vi "BodeMagnitudePlot.vi"() -> ()   [LabVIEW 2014]
uses:
  <vilib>/Analysis/NI_AALPro.lvlib
panel:
  out "XY Graph":cluster{i32, "AC estimate (Vrms)":dbl}[](graph)=[{10, "AC estimate (Vrms)"=-0.004675753198457834}, {35, "AC estimate (Vrms)"=-0.0035149121931835688}, {60, "AC estimate (Vrms)"=-0.051563979113297576}, {85, "AC estimate (Vrms)"=-0.14643905954366332}, {110, "AC estimate (Vrms)"=-0.2862310414848757}, {135, "AC estimate (Vrms)"=-0.46598201365644476}, {160, "AC estimate (Vrms)"=-0.6815881505200081}, {185, "AC estimate (Vrms)"=-0.9263195065800965}, {210, "AC estimate (Vrms)"=-1.1964263775659787}, {235, "AC estimate (Vrms)"=-1.485406346618758}, {260, "AC estimate (Vrms)"=-1.78932680664906}, {285, "AC estimate (Vrms)"=-2.1037025669360143}, {310, "AC estimate (Vrms)"=-2.424555442077878}, {335, "AC estimate (Vrms)"=-2.7502560417202444}, {360, "AC estimate (Vrms)"=-3.0771931181872194}, {385, "AC estimate (Vrms)"=-3.4039411837381777}, {410, "AC estimate (Vrms)"=-3.7283021336466176}, {435, "AC estimate (Vrms)"=-4.049588569724464}, {460, "AC estimate (Vrms)"=-4.367170083762293}, {485, "AC estimate (Vrms)"=-4.679307662238465}, {510, "AC estimate (Vrms)"=-4.98648280296608}, {535, "AC estimate (Vrms)"=-5.287209643051201}, {560, "AC estimate (Vrms)"=-5.582617535968515}, {585, "AC estimate (Vrms)"=-5.871609774751826}, {610, "AC estimate (Vrms)"=-6.154783342432669}, {635, "AC estimate (Vrms)"=-6.431856406508438}, {660, "AC estimate (Vrms)"=-6.702416154538567}, {685, "AC estimate (Vrms)"=-6.967383164412367}, {710, "AC estimate (Vrms)"=-7.2252276630895205}, {735, "AC estimate (Vrms)"=-7.478724412425297}, {760, "AC estimate (Vrms)"=-7.725316314779521}, {785, "AC estimate (Vrms)"=-7.967273470541409}, {810, "AC estimate (Vrms)"=-8.203881858765337}, {835, "AC estimate (Vrms)"=-8.434595632825712}, {860, "AC estimate (Vrms)"=-8.661455737583516}, {885, "AC estimate (Vrms)"=-8.88271571733863}, {910, "AC estimate (Vrms)"=-9.100239518286852}, {935, "AC estimate (Vrms)"=-9.312928832637102}, {960, "AC estimate (Vrms)"=-9.51985916436789}, {985, "AC estimate (Vrms)"=-9.723676817120928}, {1010, "AC estimate (Vrms)"=-9.92308680908233}, {1035, "AC estimate (Vrms)"=-10.118265706927163}, {1060, "AC estimate (Vrms)"=-10.310528942455717}, {1085, "AC estimate (Vrms)"=-10.49945287652739}, {1110, "AC estimate (Vrms)"=-10.682789281224196}, {1135, "AC estimate (Vrms)"=-10.86335084920713}, {1160, "AC estimate (Vrms)"=-11.041480017377193}, {1185, "AC estimate (Vrms)"=-11.215541236406958}, {1210, "AC estimate (Vrms)"=-11.386291463482006}, {1235, "AC estimate (Vrms)"=-11.55533757735563}, {1260, "AC estimate (Vrms)"=-11.718673081017934}, {1285, "AC estimate (Vrms)"=-11.88136948246116}, {1310, "AC estimate (Vrms)"=-12.042322604095855}, {1335, "AC estimate (Vrms)"=-12.19691149584682}, {1360, "AC estimate (Vrms)"=-12.352021455608037}, {1385, "AC estimate (Vrms)"=-12.502765768732168}, {1410, "AC estimate (Vrms)"=-12.652880465115945}, {1435, "AC estimate (Vrms)"=-12.800649157691815}, {1460, "AC estimate (Vrms)"=-12.944895119344324}, {1485, "AC estimate (Vrms)"=-13.087263149107251}, {1510, "AC estimate (Vrms)"=-13.227913974535666}, {1535, "AC estimate (Vrms)"=-13.366434802395254}, {1560, "AC estimate (Vrms)"=-13.501711703169189}, {1585, "AC estimate (Vrms)"=-13.63492997319759}, {1610, "AC estimate (Vrms)"=-13.768663430844603}, {1635, "AC estimate (Vrms)"=-13.899086027005456}, {1660, "AC estimate (Vrms)"=-14.025193743880939}, {1685, "AC estimate (Vrms)"=-14.15268151543668}, {1710, "AC estimate (Vrms)"=-14.279104082578106}, {1735, "AC estimate (Vrms)"=-14.402577876263809}, {1760, "AC estimate (Vrms)"=-14.523633716915686}, {1785, "AC estimate (Vrms)"=-14.64470374157941}, {1810, "AC estimate (Vrms)"=-14.762990967490033}, {1835, "AC estimate (Vrms)"=-14.87884715607221}, {1860, "AC estimate (Vrms)"=-14.995860488208049}, {1885, "AC estimate (Vrms)"=-15.110050634669099}, {1910, "AC estimate (Vrms)"=-15.221670884093152}, {1935, "AC estimate (Vrms)"=-15.333322732320472}, {1960, "AC estimate (Vrms)"=-15.443975891203012}, {1985, "AC estimate (Vrms)"=-15.552334841161246}, {2010, "AC estimate (Vrms)"=-15.660020622054414}]
  out "Array":cluster{"G=20*log10(Vout/Vin)":dbl, i32}[](array[cluster])=[{"G=20*log10(Vout/Vin)"=10.0, 0}, {"G=20*log10(Vout/Vin)"=35.0, 0}, {"G=20*log10(Vout/Vin)"=60.0, 0}, {"G=20*log10(Vout/Vin)"=85.0, 0}, {"G=20*log10(Vout/Vin)"=110.0, 0}, {"G=20*log10(Vout/Vin)"=135.0, 0}, {"G=20*log10(Vout/Vin)"=160.0, -1}, {"G=20*log10(Vout/Vin)"=185.0, -1}, {"G=20*log10(Vout/Vin)"=210.0, -1}, {"G=20*log10(Vout/Vin)"=235.0, -1}, {"G=20*log10(Vout/Vin)"=260.0, -2}, {"G=20*log10(Vout/Vin)"=285.0, -2}, {"G=20*log10(Vout/Vin)"=310.0, -2}, {"G=20*log10(Vout/Vin)"=335.0, -3}, {"G=20*log10(Vout/Vin)"=360.0, -3}, {"G=20*log10(Vout/Vin)"=385.0, -3}, {"G=20*log10(Vout/Vin)"=410.0, -4}, {"G=20*log10(Vout/Vin)"=435.0, -4}, {"G=20*log10(Vout/Vin)"=460.0, -4}, {"G=20*log10(Vout/Vin)"=485.0, -5}, {"G=20*log10(Vout/Vin)"=510.0, -5}, {"G=20*log10(Vout/Vin)"=535.0, -5}, {"G=20*log10(Vout/Vin)"=560.0, -6}, {"G=20*log10(Vout/Vin)"=585.0, -6}, {"G=20*log10(Vout/Vin)"=610.0, -6}, {"G=20*log10(Vout/Vin)"=635.0, -6}, {"G=20*log10(Vout/Vin)"=660.0, -7}, {"G=20*log10(Vout/Vin)"=685.0, -7}, {"G=20*log10(Vout/Vin)"=710.0, -7}, {"G=20*log10(Vout/Vin)"=735.0, -7}, {"G=20*log10(Vout/Vin)"=760.0, -8}, {"G=20*log10(Vout/Vin)"=785.0, -8}, {"G=20*log10(Vout/Vin)"=810.0, -8}, {"G=20*log10(Vout/Vin)"=835.0, -8}, {"G=20*log10(Vout/Vin)"=860.0, -9}, {"G=20*log10(Vout/Vin)"=885.0, -9}, {"G=20*log10(Vout/Vin)"=910.0, -9}, {"G=20*log10(Vout/Vin)"=935.0, -9}, {"G=20*log10(Vout/Vin)"=960.0, -10}, {"G=20*log10(Vout/Vin)"=985.0, -10}, {"G=20*log10(Vout/Vin)"=1010.0, -10}, {"G=20*log10(Vout/Vin)"=1035.0, -10}, {"G=20*log10(Vout/Vin)"=1060.0, -10}, {"G=20*log10(Vout/Vin)"=1085.0, -10}, {"G=20*log10(Vout/Vin)"=1110.0, -11}, {"G=20*log10(Vout/Vin)"=1135.0, -11}, {"G=20*log10(Vout/Vin)"=1160.0, -11}, {"G=20*log10(Vout/Vin)"=1185.0, -11}, {"G=20*log10(Vout/Vin)"=1210.0, -11}, {"G=20*log10(Vout/Vin)"=1235.0, -12}, {"G=20*log10(Vout/Vin)"=1260.0, -12}, {"G=20*log10(Vout/Vin)"=1285.0, -12}, {"G=20*log10(Vout/Vin)"=1310.0, -12}, {"G=20*log10(Vout/Vin)"=1335.0, -12}, {"G=20*log10(Vout/Vin)"=1360.0, -12}, {"G=20*log10(Vout/Vin)"=1385.0, -13}, {"G=20*log10(Vout/Vin)"=1410.0, -13}, {"G=20*log10(Vout/Vin)"=1435.0, -13}, {"G=20*log10(Vout/Vin)"=1460.0, -13}, {"G=20*log10(Vout/Vin)"=1485.0, -13}, {"G=20*log10(Vout/Vin)"=1510.0, -13}, {"G=20*log10(Vout/Vin)"=1535.0, -13}, {"G=20*log10(Vout/Vin)"=1560.0, -14}, {"G=20*log10(Vout/Vin)"=1585.0, -14}, {"G=20*log10(Vout/Vin)"=1610.0, -14}, {"G=20*log10(Vout/Vin)"=1635.0, -14}, {"G=20*log10(Vout/Vin)"=1660.0, -14}, {"G=20*log10(Vout/Vin)"=1685.0, -14}, {"G=20*log10(Vout/Vin)"=1710.0, -14}, {"G=20*log10(Vout/Vin)"=1735.0, -14}, {"G=20*log10(Vout/Vin)"=1760.0, -15}, {"G=20*log10(Vout/Vin)"=1785.0, -15}, {"G=20*log10(Vout/Vin)"=1810.0, -15}, {"G=20*log10(Vout/Vin)"=1835.0, -15}, {"G=20*log10(Vout/Vin)"=1860.0, -15}, {"G=20*log10(Vout/Vin)"=1885.0, -15}, {"G=20*log10(Vout/Vin)"=1910.0, -15}, {"G=20*log10(Vout/Vin)"=1935.0, -15}, {"G=20*log10(Vout/Vin)"=1960.0, -15}, {"G=20*log10(Vout/Vin)"=1985.0, -16}, {"G=20*log10(Vout/Vin)"=2010.0, -16}]
  out "error out":errorcluster={"status"=FALSE, "code"=200015, "source"="DAQmx Write (Analog 1D Wfm NChan NSamp).vi:6390002"}
  # "Frequency (Hz)"
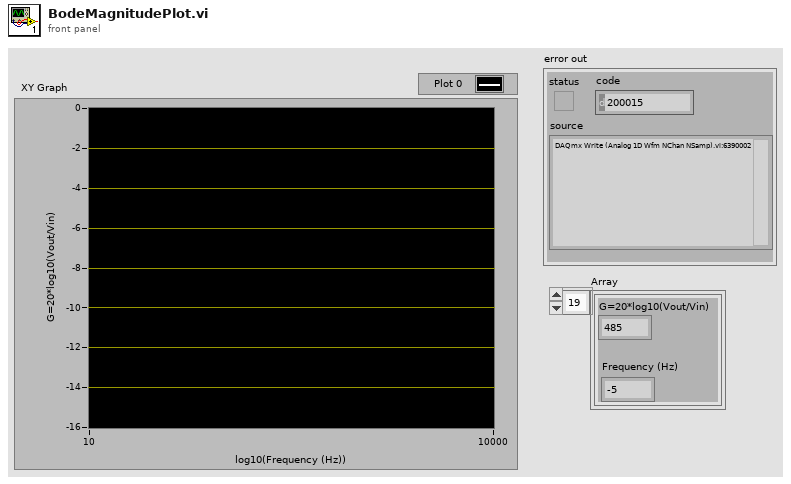
[diagram p1: front panel]
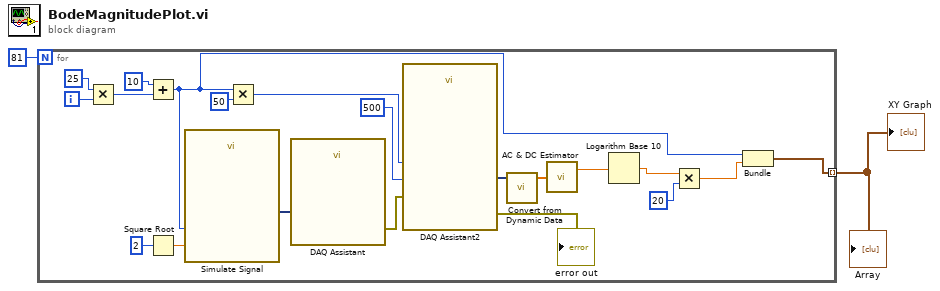
[diagram p0: block diagram]
diagram:
  n1 = for {
    N: 81 -> [_]
    tunnel: [w9] -> w1 mode=indexing
    i -> [w22]
    n2 = Multiply(x=25, y=w22) -> (x*y=w20:i32)
    n3 = Add(x=10, y=w20) -> (x+y=w7:i32)
    n4 = Square Root(x=2) -> (sqrt(x)=w17:dbl)
    n5 = call "Simulate Signal"("Frequency"=w7, "Amplitude"=w17) -> ("Sine"=w16:dynamicdata)  [unwired: 12 in, 1 out]
    n6 = Multiply(x=w7, y=50) -> (x*y=w13:i32)
    n7 = call "DAQ Assistant"("data"=w16) -> ("error out"=w15:errorcluster)  [unwired: 16 in, 2 out]
    n8 = call "DAQ Assistant2"("rate"=w13, "number of samples"=500, "error in"=w15) -> ("data"=w11:dynamicdata, "error out"=→"error out":errorcluster)  [unwired: 14 in, 1 out]
    n9 = call "Convert from Dynamic Data"("Dynamic Data Type"=w11) -> ("Array"=w10:dbl[])  [unwired: 3 in]
    n10 = call <vilib>:"AC & DC Estimator.vi"("Signal (V)"=w10) -> ("AC estimate (Vrms)"=w6:dbl)  [unwired: 1 out]
    n11 = Logarithm Base 10(1:w6) -> (0:w4:dbl)
    n12 = Multiply(x=w4, y=20) -> (x*y=w3:dbl)
    n13 = Bundle(w7, w3) -> (w9:cluster{i32, dbl})  [unwired: 1 in]
  }
  "Array" <- w1
  "XY Graph" <- w1
